vi "SNF_Digital.vi"() -> ()   [LabVIEW 2017]
uses:
  Users/Darcy/Documents/LabVIEW Data/MathScriptVIs/MCStatic_38597428832_1f828b6118eee4aae6c26f87bca7dc42.vi
  <instcachedir>/0/MCStatic_38597428832_1f828b6118eee4aae6c26f87bca7dc42_D4E3D0E3241540FEBE7742005F22DD6C.lvgen/MCStatic_38597428832_1f828b6118eee4aae6c26f87bca7dc42_D4E3D0E3241540FEBE7742005F22DD6C_000.vi
  <vilib>/imath/engines/lvmath2/RunTimeEngine/IndexRead/NIMS V(S).vi
  <instcachedir>/0/NIMS V(S)_0488751826AF41519A22953C041130DC.lvgen/NIMS V(S)_0488751826AF41519A22953C041130DC_000.vi
  <vilib>/imathl/engines/lvmath/Functions/Error Handling/Create Error.vi
  <vilib>/imath/engines/lvmath2/RunTimeEngine/NodeEndStatement/NIMS_NodeEndStatement_Output.vi
  <instcachedir>/0/NIMS_NodeEndStatement_Output_53EC0D466D134D7ABD903AC30B43404B.lvgen/NIMS_NodeEndStatement_Output_53EC0D466D134D7ABD903AC30B43404B_001.vi
  <instcachedir>/0/NIMS_NodeEndStatement_Output_53EC0D466D134D7ABD903AC30B43404B.lvgen/NIMS_NodeEndStatement_Output_53EC0D466D134D7ABD903AC30B43404B_005.vi
  <vilib>/imath/engines/lvmath2/RunTimeEngine/ErrorHandling/NIMS_Finalize Error.vi
  <vilib>/Utility/file.llb/Read Delimited Spreadsheet (DBL).vi
  Users/Darcy/Documents/LabVIEW Data/reactor_power.m
  Users/Darcy/Documents/LabVIEW Data/long_term_power.m
  Users/Darcy/Documents/LabVIEW Data/power_function.m
  Users/Darcy/Documents/LabVIEW Data/short_term_power.m
panel:
  in  "CRsteady":dbl=50.0 format="%#_13g"
  in  "CRamp":dbl=200.0
  in  "power":dbl=50.0 format="%#_13g"
  in  "P_max: 100":dbl=200.0
  in  "P_min: 1":dbl=1.0
  out "ST Avg.":dbl
  out "Coolant Temp":dbl(slide) scale=0.0..100.0
  out "Fuel Temp":dbl(slide) scale=0.0..100.0
  out "BT Avg.":dbl
  out "CX Avg.":dbl
  in  "Input Length":dbl
  out "Iterations":dbl
  in  "?":bool
  in  "?":bool
  out "Array":dbl[](array[numeric])
  in  "INPUT/MANUAL":bool
  in  "Load Power Profile":bool
  in  "Dyn. Control Rod Profile File":path
  in  "?":bool
  in  "Equilibrium T_Coolant\nFHR: 100":dbl=100.0
  in  "Equilibrium T_Fuel\nFHR: 100":dbl=100.0
  in  "Coolant Feedback Coef\nFHR: -2.1":dbl=-2.1
  in  "Fuel Feedback Coef\nFHR: -6.7":dbl=-6.7
  in  "CRW Coef":dbl=0.005
  in  "CRW Constant":dbl=0.997
  in  "beta\nFHR: 0.0065":dbl=0.0065
  in  "Lambda\nFHR: 5.02e-4":dbl=0.000502
  in  "lambda\nFHR: 0.0785":dbl=0.0785
  out "Net Reactivity":dbl
  out "Rod Reactivity":dbl
  out "Rod 1 In":dbl(slide)
  out "Rod 1 Out":dbl(slide) scale=0.0..1.0
  out "?":dbl(slide) scale=1.0..100.0
  out "Net Amount Rod Out":dbl
  out "Power [W]":dbl
  in  "SCRAM":bool
  out "Power":dbl(graph)
  out "Resolution 1":dbl=0.05
  out "Control Rod 1 Out":dbl=0.6
  in  "STOP TOGGLE":bool
  # "Neutronics"
  # "Control Rod Worth (CRW)"
  # "Outside Core"
  # "Inside Core"
  # "Temperature Feedback"
  # "Fine"
  # "Input"
  # "Manual"
  # "Coarse"
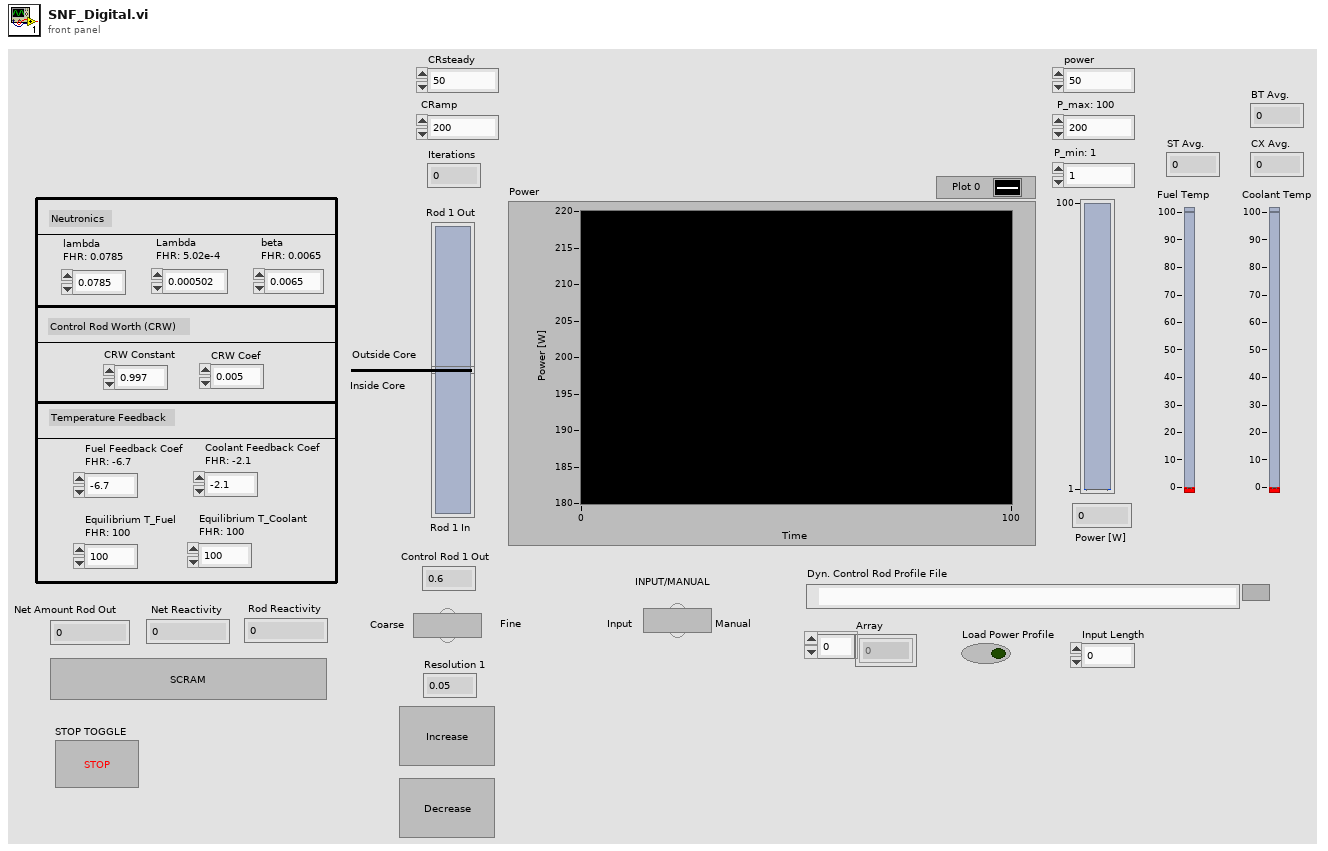
[diagram p1: front panel]
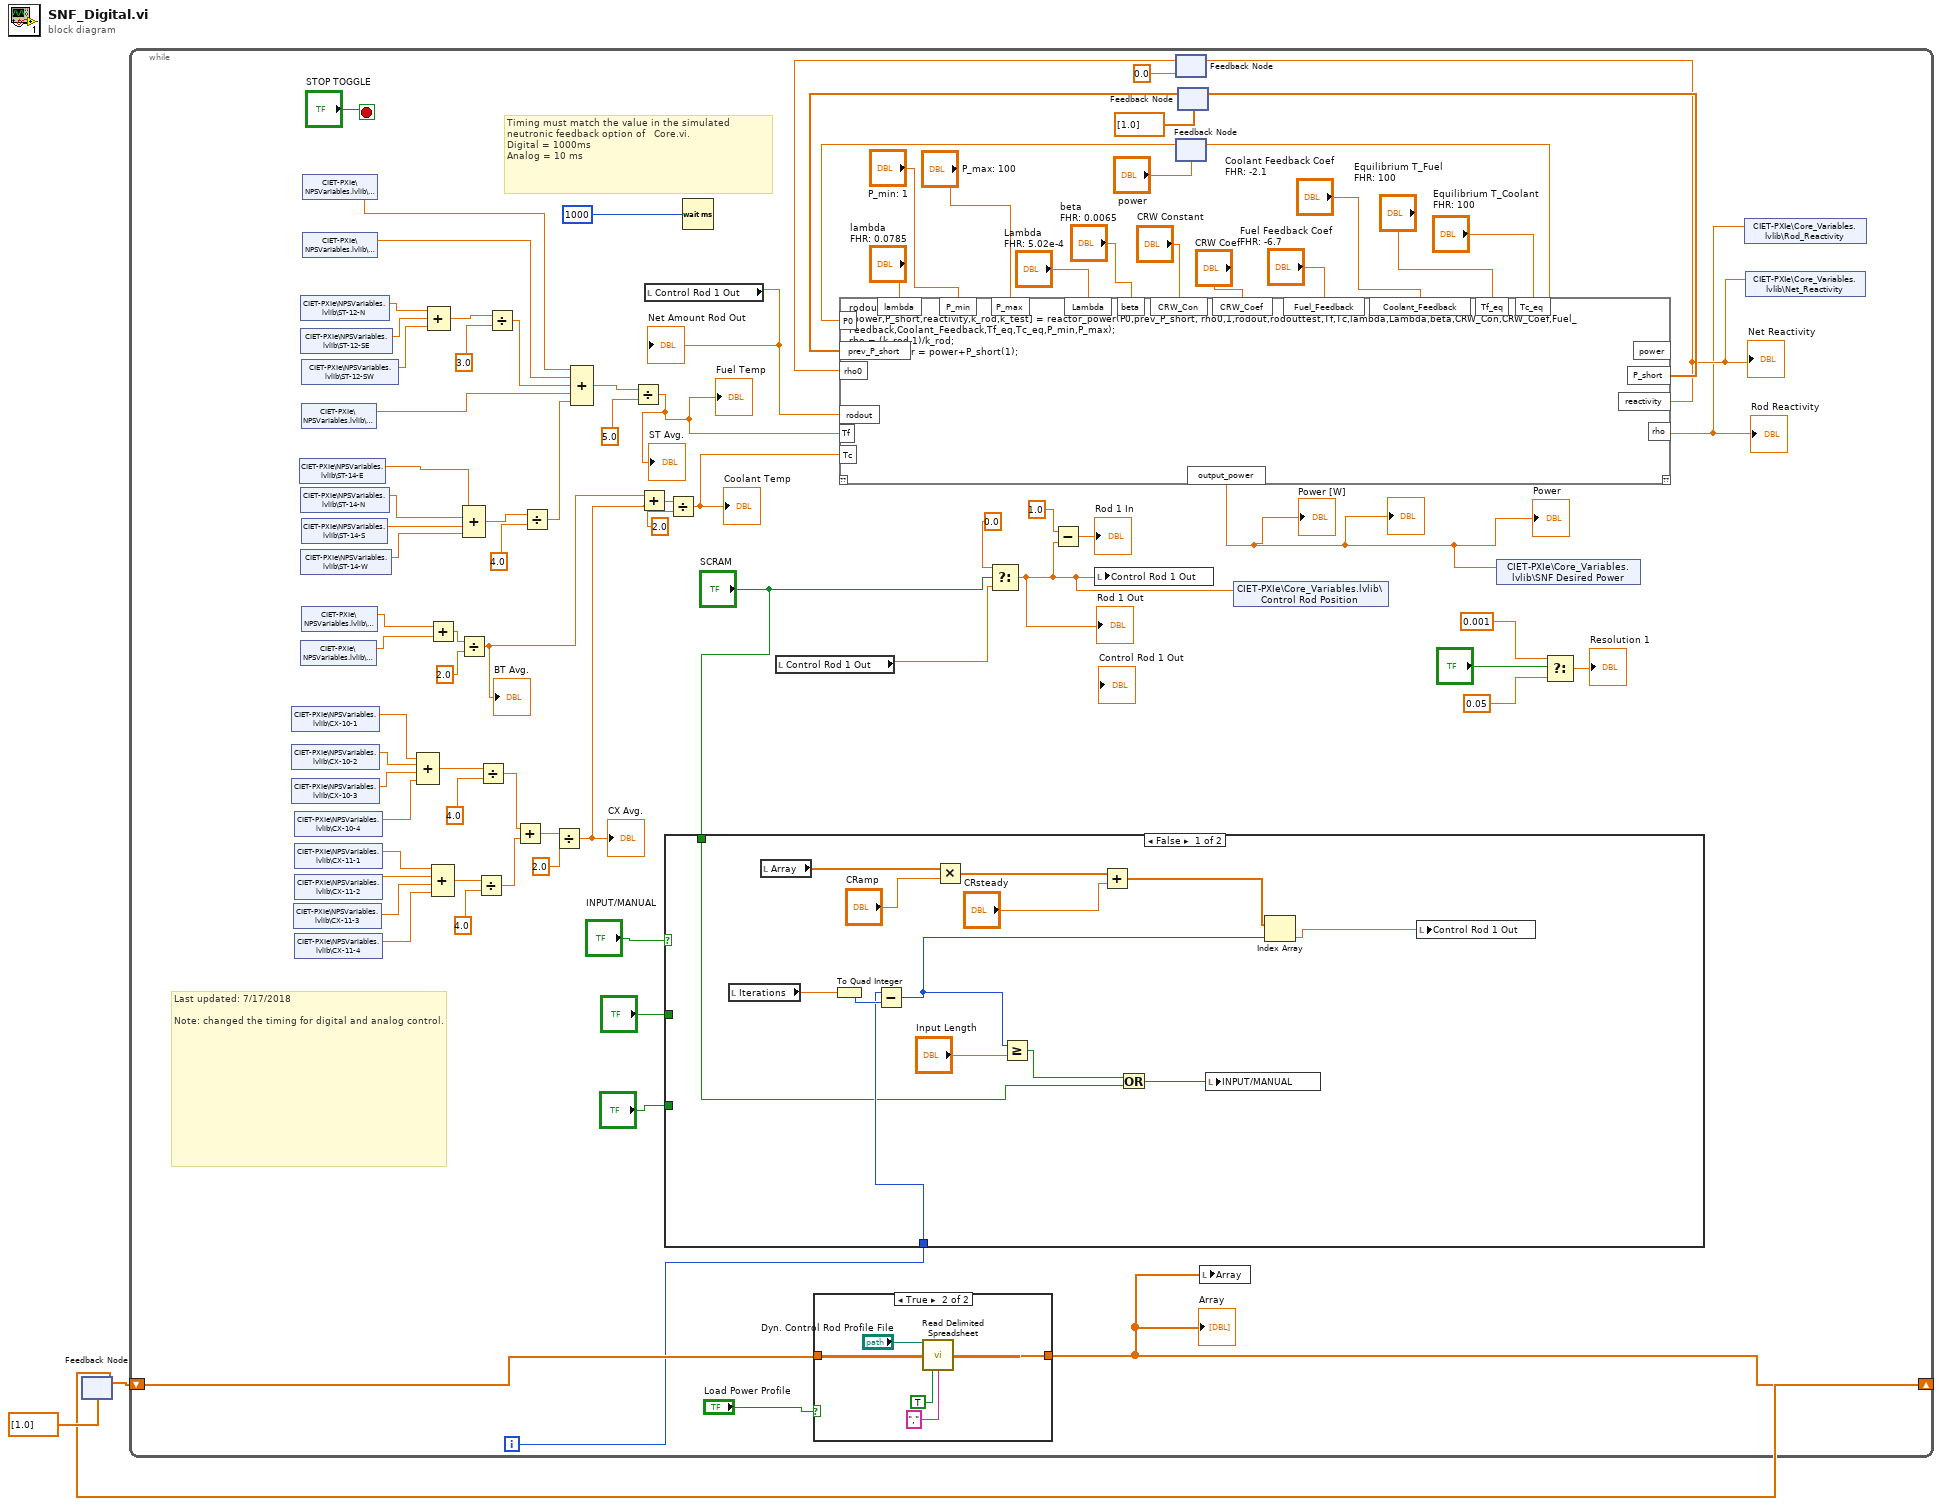
[diagram p0: block diagram]
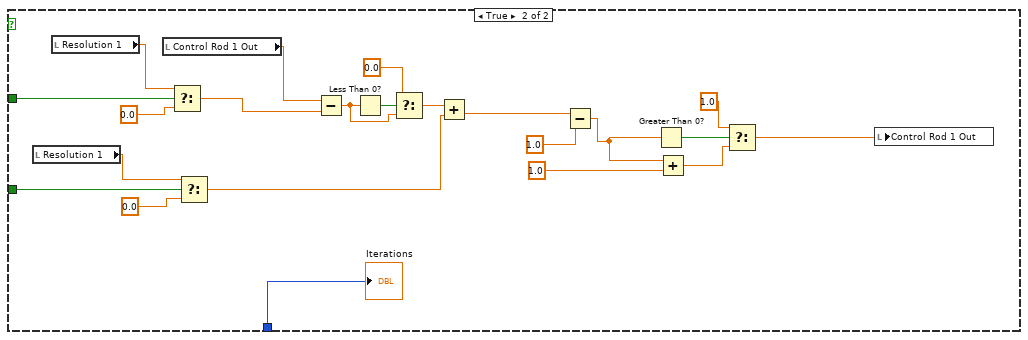
[diagram p2: hidden frame]
diagram:
  n1 = feedback #1(dbl[] [1.0] ("P_short")) -> (w3:dbl[])
  n2 = while {
    shift-right: [w61] -> w1
    shift-left: w3 -> [w62]
    i -> [w56]
    stop <- "STOP TOGGLE" stop-if-true
    # "Last updated: 7/17/2018\n\nNote: changed the timing for digital and analog control."
    # "Timing must match the value in the simulated neutronic feedback option of   Core.vi. \nDigital = 1000ms \nAnalog = 10 ms"
    n3 = shared-variable "CIET-PXIe\\NPSVariables.lvlib\\CX-10-1"() -> (w20:sgl)  [unwired: 1 in, 1 out]
    n4 = shared-variable "CIET-PXIe\\NPSVariables.lvlib\\CX-10-2"() -> (w19:sgl)  [unwired: 1 in, 1 out]
    n5 = shared-variable "CIET-PXIe\\NPSVariables.lvlib\\CX-10-3"() -> (w18:sgl)  [unwired: 1 in, 1 out]
    n6 = shared-variable "CIET-PXIe\\NPSVariables.lvlib\\CX-11-3"() -> (w14:sgl)  [unwired: 1 in, 1 out]
    n7 = shared-variable "CIET-PXIe\\NPSVariables.lvlib\\CX-10-4"() -> (w17:sgl)  [unwired: 1 in, 1 out]
    n8 = shared-variable "CIET-PXIe\\NPSVariables.lvlib\\CX-11-1"() -> (w16:sgl)  [unwired: 1 in, 1 out]
    n9 = shared-variable "CIET-PXIe\\NPSVariables.lvlib\\CX-11-2"() -> (w15:sgl)  [unwired: 1 in, 1 out]
    n10 = shared-variable "CIET-PXIe\\NPSVariables.lvlib\\CX-11-4"() -> (w13:sgl)  [unwired: 1 in, 1 out]
    n11 = shared-variable "CIET-PXIe\\NPSVariables.lvlib\\ST-14-E"() -> (w36:sgl)  [unwired: 1 in, 1 out]
    n12 = shared-variable "CIET-PXIe\\NPSVariables.lvlib\\ST-12-N"() -> (w43:sgl)  [unwired: 1 in, 1 out]
    n13 = shared-variable "CIET-PXIe\\NPSVariables.lvlib\\ST-12-SE"() -> (w42:sgl)  [unwired: 1 in, 1 out]
    n14 = shared-variable "CIET-PXIe\\NPSVariables.lvlib\\ST-14-N"() -> (w35:sgl)  [unwired: 1 in, 1 out]
    n15 = shared-variable "CIET-PXIe\\NPSVariables.lvlib\\ST-14-W"() -> (w33:sgl)  [unwired: 1 in, 1 out]
    n16 = shared-variable "CIET-PXIe\\NPSVariables.lvlib\\BT-12"() -> (w50:sgl)  [unwired: 1 in, 1 out]
    n17 = shared-variable "CIET-PXIe\\NPSVariables.lvlib\\ST-12-SW"() -> (w41:sgl)  [unwired: 1 in, 1 out]
    n18 = shared-variable "CIET-PXIe\\NPSVariables.lvlib\\ST-13"() -> (w39:sgl)  [unwired: 1 in, 1 out]
    n19 = shared-variable "CIET-PXIe\\NPSVariables.lvlib\\ST-14-S"() -> (w34:sgl)  [unwired: 1 in, 1 out]
    n20 = shared-variable "CIET-PXIe\\NPSVariables.lvlib\\BT-11"() -> (w51:sgl)  [unwired: 1 in, 1 out]
    n21 = shared-variable "CIET-PXIe\\NPSVariables.lvlib\\ST-10"() -> (w49:sgl)  [unwired: 1 in, 1 out]
    n22 = shared-variable "CIET-PXIe\\NPSVariables.lvlib\\ST-11"() -> (w48:sgl)  [unwired: 1 in, 1 out]
    n23 = Compound Arithmetic op=ADD(w20, w19, w18, w17) -> (w26:sgl)
    n24 = Compound Arithmetic op=ADD(w43, w42, w41) -> (w45:sgl)
    n25 = Add(x=w51, y=w50) -> (x+y=w53:sgl)
    n26 = Compound Arithmetic op=ADD(w16, w15, w14, w13) -> (w24:sgl)
    n27 = Divide(x=w53, y=2.0) -> (x/y=w30:dbl)
    "BT Avg." <- w30
    n28 = Compound Arithmetic op=ADD(w36, w35, w34, w33) -> (w38:sgl)
    n29 = Divide(x=w24, y=4.0) -> (x/y=w21:dbl)
    n30 = Divide(x=w26, y=4.0) -> (x/y=w22:dbl)
    n31 = Divide(x=w45, y=3.0) -> (x/y=w40:dbl)
    n32 = Add(x=w22, y=w21) -> (x+y=w55:dbl)
    n33 = Divide(x=w38, y=4.0) -> (x/y=w32:dbl)
    n34 = Divide(x=w55, y=2.0) -> (x/y=w29:dbl)
    "CX Avg." <- w29
    n35 = Compound Arithmetic op=ADD(w49, w48, w40, w39, w32) -> (w47:dbl)
    n36 = Divide(x=w47, y=5.0) -> (x/y=w12:dbl)
    "Fuel Temp" <- w12
    "ST Avg." <- w12
    n37 = Add(x=w30, y=w29) -> (x+y=w28:dbl)
    n38 = local read "Control Rod 1 Out"() -> (w64:dbl)
    "Net Amount Rod Out" <- w64
    n39 = case shown="False" "INPUT/MANUAL" {
      tunnel: "?" -> [_ w107]
      tunnel: "?" -> [_ w106]
      tunnel: w56 -> [w99 w105]
      tunnel: "SCRAM" -> [w97 _]
      frame False {
        n40 = local read "Iterations"() -> (w101:dbl)
        n41 = local read "Array"() -> (w94:dbl[])
        n42 = To Quad Integer(1:w101) -> (0:w100:i64)
        n43 = Subtract(x=w99, y=w100) -> (x-y=w102:i64)
        n44 = Multiply(x=w94, y="CRamp") -> (x*y=w92:dbl[])
        n45 = Greater Or Equal?(x=w102, y="Input Length") -> (x >= y?=w98:bool)
        n46 = Add(x=w92, y="CRsteady") -> (x+y=w90:dbl[])
        n47 = Or(x=w98, y=w97) -> (x .or. y?=w96:bool)
        n48 = local write "INPUT/MANUAL"(w96) -> ()
        n49 = Index Array(array=w90, index=w102) -> (element=w95:dbl)
        n50 = local write "Control Rod 1 Out"(w95) -> ()
      }
      frame True {
        n51 = local read "Resolution 1"() -> (w123:dbl)
        n52 = local read "Resolution 1"() -> (w125:dbl)
        n53 = local read "Control Rod 1 Out"() -> (w121:dbl)
        n54 = Select(t=w125, s=w107, f=0.0) -> (s? t:f=w120:dbl)
        n55 = Select(t=w123, s=w106, f=0.0) -> (s? t:f=w108:dbl)
        n56 = Subtract(x=w121, y=w120) -> (x-y=w118:dbl)
        n57 = Less Than 0?(x=w118) -> (x < 0?=w119:bool)
        n58 = Select(t=0.0, s=w119, f=w118) -> (s? t:f=w116:dbl)
        n59 = Add(x=w116, y=w108) -> (x+y=w115:dbl)
        n60 = Subtract(x=w115, y=1.0) -> (x-y=w111:dbl)
        n61 = Greater Than 0?(x=w111) -> (x > 0?=w113:bool)
        n62 = Add(x=w111, y=1.0) -> (x+y=w110:dbl)
        n63 = Select(t=1.0, s=w113, f=w110) -> (s? t:f=w104:dbl)
        n64 = local write "Control Rod 1 Out"(w104) -> ()
        "Iterations" <- w105
      }
    }
    n65 = Divide(x=w28, y=2.0) -> (x/y=w27:dbl)
    "Coolant Temp" <- w27
    n66 = Wait (ms)(milliseconds to wait=u32 1000) -> ()  [unwired: 1 out]
    n67 = local read "Control Rod 1 Out"() -> (w57:dbl)
    n68 = case shown="True" "Load Power Profile" {
      tunnel: [w126 w127] -> w61
      tunnel: w62 -> [w126 _]
      frame False {
      }
      frame True {
        n69 = call-poly <vilib>:"Read Delimited Spreadsheet.vi"("file path (dialog if empty)"="Dyn. Control Rod Profile File", "transpose? (F)"=TRUE, "delimiter (\\t)"="," ("delimiter (\\t)")) -> ("first row"=w127:dbl[])  [unwired: 7 in, 5 out]
      }
    }
    "Array" <- w61
    n70 = Select(t=0.0, s="SCRAM", f=w57) -> (s? t:f=w7:dbl)
    "Rod 1 Out" <- w7
    n71 = Subtract(x=1.0, y=w7) -> (x-y=→"Rod 1 In":dbl)
    n72 = local write "Control Rod 1 Out"(w7) -> ()
    n73 = feedback #2(0.0 ("reactivity")) -> (w81:dbl)
    n74 = feedback #3("power") -> (w84:dbl)
    n75 = feedback #4(dbl[] [1.0] ("P_short")) -> (w82:dbl[])
    n76 = mathscript code="rodouttest = 0;\n[power,P_short,reactivity,k_rod,k_test] = reactor_power(P0,prev_P_short, rho0,1,rodout,rodouttest,Tf,Tc,lambda,Lambda,beta,CRW_Con,CRW_Coef,Fuel_Feedback,Coolant_Feedback,Tf_eq,Tc_eq,P_min,P_max);\nrho = (k_rod-1)/k_rod;\noutput_power = power+P_short(1);"("rodout"=w64, "P0"=w84, "prev_P_short"=w82, "rho0"=w81, "Tf"=w12, "Tc"=w27, "lambda"="lambda\nFHR: 0.0785", "Lambda"="Lambda\nFHR: 5.02e-4", "beta"="beta\nFHR: 0.0065", "CRW_Con"="CRW Constant", "CRW_Coef"="CRW Coef", "Fuel_Feedback"="Fuel Feedback Coef\nFHR: -6.7", "Coolant_Feedback"="Coolant Feedback Coef\nFHR: -2.1", "Tf_eq"="Equilibrium T_Fuel\nFHR: 100", "Tc_eq"="Equilibrium T_Coolant\nFHR: 100", "P_max"="P_max: 100", "P_min"="P_min: 1") -> ("power"=w85:dbl, "P_short"=w83:dbl[], "reactivity"=w6:dbl, "output_power"=w8:dbl, "rho"=w5:dbl)  [unwired: 1 in, 1 out]
    "Power" <- w8
    "Power [W]" <- w8
    "?" <- w8
    "Rod Reactivity" <- w5
    "Net Reactivity" <- w6
    n77 = feedback-in #2(w6) -> ()
    n78 = feedback-in #3(w85) -> ()
    n79 = feedback-in #4(w83) -> ()
    n80 = local write "Array"(w61) -> ()
    n81 = shared-variable "CIET-PXIe\\Core_Variables.lvlib\\Control Rod Position"(w7) -> ()  [unwired: 1 in, 1 out]
    n82 = shared-variable "CIET-PXIe\\Core_Variables.lvlib\\SNF Desired Power"(w8) -> ()  [unwired: 1 in, 1 out]
    n83 = Select(t=0.001, s="?", f=0.05) -> (s? t:f=→"Resolution 1":dbl)
    n84 = shared-variable "CIET-PXIe\\Core_Variables.lvlib\\Rod_Reactivity"(w5) -> ()  [unwired: 1 in, 1 out]
    n85 = shared-variable "CIET-PXIe\\Core_Variables.lvlib\\Net_Reactivity"(w6) -> ()  [unwired: 1 in, 1 out]
  }
  n86 = feedback-in #1(w1) -> ()
